vi "TestOpmuxa.vi"() -> ()   [LabVIEW 2013]
uses:
  Multiplexer_Opmux.lvclass
panel:
  out "BufferOut 2":string
  out "BufferOut":string
  out "DevState":bool
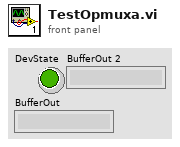
[diagram p1: front panel]
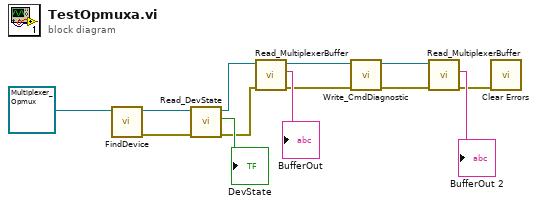
[diagram p0: block diagram]
diagram:
  n1 = call-dynamic "FindDevice.vi"("Multiplexer_Opmux in"=refnum<class "Multiplexer_Opmux.lvclass"> refnum ("Multiplexer_Opmux.lvclass")) -> ("error out"=w2:errorcluster, "Multiplexer_Opmux out"=w12:refnum<class "Multiplexer_Opmux.lvclass">)  [unwired: 8 in, 1 out]
  n2 = call-dynamic "Read_DevState.vi"("error in (no error)"=w2, "Multiplexer_Opmux in"=w12) -> ("error out"=w5:errorcluster, "DevState"=→"DevState":bool, "Multiplexer_Opmux out"=w10:refnum<class "Multiplexer_Opmux.lvclass">)  [unwired: 7 in]
  n3 = call-dynamic "Read_MultiplexerBuffer.vi"("error in (no error)"=w5, "Multiplexer_Opmux in"=w10) -> ("error out"=w4:errorcluster, "BufferOut"=→"BufferOut":string, "Multiplexer_Opmux out"=w8:refnum<class "Multiplexer_Opmux.lvclass">)  [unwired: 7 in]
  n4 = call-dynamic "Write_CmdDiagnostic.vi"("error in (no error)"=w4, "Multiplexer_Opmux in"=w8) -> ("error out"=w3:errorcluster, "Multiplexer_Opmux out"=w7:refnum<class "Multiplexer_Opmux.lvclass">)  [unwired: 8 in]
  n5 = call-dynamic "Read_MultiplexerBuffer.vi"("error in (no error)"=w3, "Multiplexer_Opmux in"=w7) -> ("error out"=w1:errorcluster, "BufferOut"=→"BufferOut 2":string)  [unwired: 7 in, 1 out]
  n6 = call <vilib>:"Clear Errors.vi"("error in (no error)"=w1) -> ()  [unwired: 6 in, 1 out]
